vi "Read Jump To.vi"(8 "error in (no error)":errorcluster, 11 "Conditional Jump Step in":refnum<class "Conditional Jump Step.lvclass">) -> (0 "error out":errorcluster, 2 "Jump To":i32, 3 "Conditional Jump Step out":refnum<class "Conditional Jump Step.lvclass">)   [LabVIEW 2015, in "Conditional Jump Step.lvclass"]
uses:
  Conditional Jump Step.lvclass
  Conditional Jump Step.lvclass/Conditional Jump Step.ctl
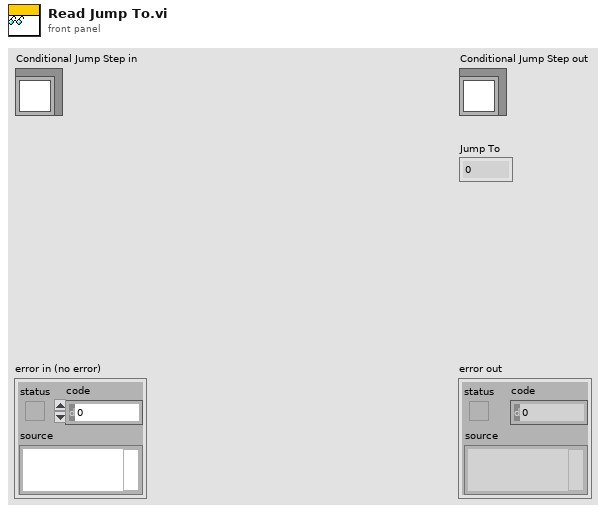
[diagram p1: front panel]
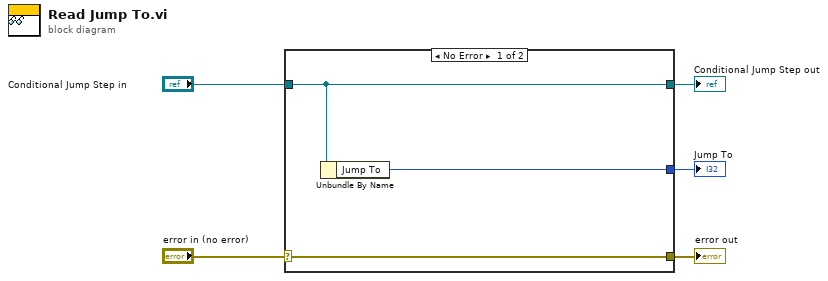
[diagram p0: block diagram]
diagram:
  n1 = case shown="No Error" "error in (no error)" {
    selector: "error in (no error)" -> [w8 w9]
    tunnel: [w8 w9] -> w4
    tunnel: [w7 w10] -> w2
    tunnel: "Conditional Jump Step in" -> [w7 w10]
    tunnel: [w6 _] -> w1
    frame No Error {
      n2 = Unbundle By Name(w7) -> ("Jump To"=w6:i32)
    }
    frame Error {
    }
  }
  "error out" <- w4
  "Conditional Jump Step out" <- w2
  "Jump To" <- w1
